vi "GetPlotConfigurations.vi"(5 "plots":refnum<class "Plot.lvclass">[](array[class])) -> (4 "plots cfg":T1[](array[typedef]))   [LabVIEW 2014, in "Raspberry Pi Compatible Compiler for LabVIEW.lvlib" / "PythonConverter_GUI.lvclass"]
uses:
  PythonConverter_GUI.lvclass
  PythonConfiguration/TypeDefs/ItemTD.ctl
  VI Interpreter/Classes/Plot/Plot.lvclass
  VI Interpreter/Classes/Plot/Plot.lvclass/Plot.ctl
  PythonConfiguration/PythonConfiguration.lvclass
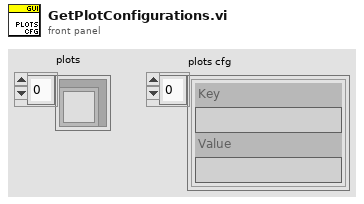
[diagram p1: front panel]
types:
  T1 = typedef "Raspberry Pi Compatible Compiler for LabVIEW.lvlib/PythonConfiguration.lvclass/ItemTD.ctl" = cluster{"Key":string, "Value":string}
  T2 = cluster{"Plot Color":u32, "Plot Interpolation":u8, "Point Style":u8, "Line Style":u8, "Fill/Pt. Color":u32, "Line Width":u8, "Bar Plot Style":u8, "Fill To":i16}
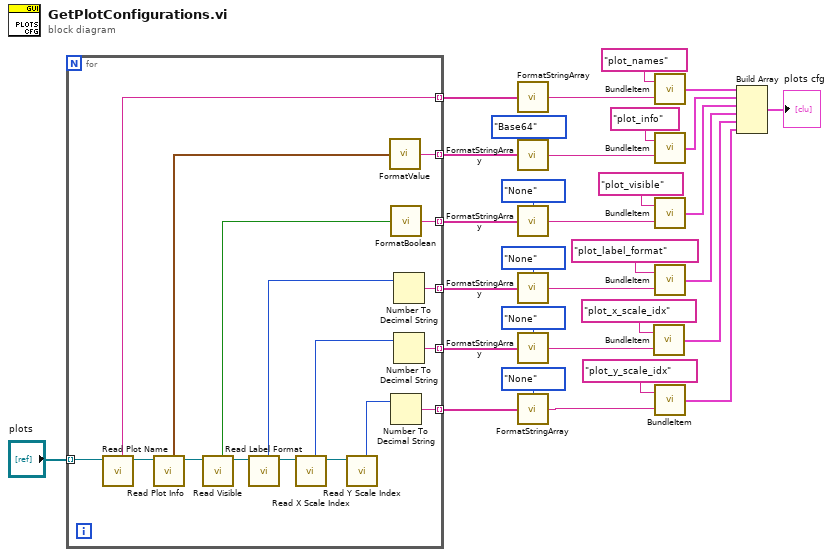
[diagram p0: block diagram]
diagram:
  n1 = for {
    tunnel: "plots" -> [w48] mode=indexing
    tunnel: [w42] -> w30 mode=indexing
    tunnel: [w40] -> w29 mode=indexing
    tunnel: [w38] -> w27 mode=indexing
    tunnel: [w36] -> w24 mode=indexing
    tunnel: [w34] -> w22 mode=indexing
    tunnel: [w32] -> w20 mode=indexing
    n2 = call "Read Plot Name.vi"("Plot in"=w48) -> ("Plot out"=w47:refnum<class "Plot.lvclass">, "Plot Name"=w42:string)  [unwired: 7 in]
    n3 = call "Read Plot Info.vi"("Plot in"=w47) -> ("Plot out"=w46:refnum<class "Plot.lvclass">, "Plot Info"=w41:T2)  [unwired: 7 in]
    n4 = call "Read Visible.vi"("Plot in"=w46) -> ("Plot out"=w45:refnum<class "Plot.lvclass">, "Visible"=w39:bool)  [unwired: 7 in]
    n5 = call "Read Label Format.vi"("Plot in"=w45) -> ("Plot out"=w44:refnum<class "Plot.lvclass">, "Label Format"=w37:u8)  [unwired: 7 in]
    n6 = call "Read X Scale Index.vi"("Plot in"=w44) -> ("Plot out"=w43:refnum<class "Plot.lvclass">, "X Scale Index"=w35:u32)  [unwired: 7 in]
    n7 = call "Read Y Scale Index.vi"("Plot in"=w43) -> ("Y Scale Index"=w33:u32)  [unwired: 7 in, 1 out]
    n8 = call "FormatValue.vi"("value"=w41) -> ("value"=w40:string)
    n9 = call "FormatBoolean.vi"("boolean"=w39) -> ("value"=w38:string)
    n10 = Number To Decimal String(number=w33) -> (decimal integer string=w32:string)  [unwired: 1 in]
    n11 = Number To Decimal String(number=w37) -> (decimal integer string=w36:string)  [unwired: 1 in]
    n12 = Number To Decimal String(number=w35) -> (decimal integer string=w34:string)  [unwired: 1 in]
  }
  n13 = call "FormatStringArray.vi"("strings"=w30) -> ("value"=w19:string)  [unwired: 1 in]
  n14 = call "FormatStringArray.vi"("strings"=w29, "string encoding"=enum16{"None", "Base64"}."Base64") -> ("value"=w16:string)
  n15 = call "FormatStringArray.vi"("strings"=w27, "string encoding"=enum16{"None", "Base64"}."None") -> ("value"=w14:string)
  n16 = call "FormatStringArray.vi"("strings"=w24, "string encoding"=enum16{"None", "Base64"}."None") -> ("value"=w12:string)
  n17 = call "FormatStringArray.vi"("strings"=w22, "string encoding"=enum16{"None", "Base64"}."None") -> ("value"=w10:string)
  n18 = call "FormatStringArray.vi"("strings"=w20, "string encoding"=enum16{"None", "Base64"}."None") -> ("value"=w8:string)
  n19 = call "BundleItem.vi"("Value"=w10, "Key"="plot_x_scale_idx") -> ("Item"=w3:T1)
  n20 = call "BundleItem.vi"("Value"=w19, "Key"="plot_names") -> ("Item"=w7:T1)
  n21 = call "BundleItem.vi"("Value"=w16, "Key"="plot_info") -> ("Item"=w6:T1)
  n22 = call "BundleItem.vi"("Value"=w14, "Key"="plot_visible") -> ("Item"=w5:T1)
  n23 = call "BundleItem.vi"("Value"=w12, "Key"="plot_label_format") -> ("Item"=w4:T1)
  n24 = call "BundleItem.vi"("Value"=w8, "Key"="plot_y_scale_idx") -> ("Item"=w2:T1)
  n25 = Build Array(w7, w6, w5, w4, w3, w2) -> (→"plots cfg":T1[])
